vi "Do.vi"(8 "error in":errorcluster, 10 "Actor in":refnum<class "Actor.lvclass">, 11 "DS Reply Msg in":refnum<class "Reply Msg DataSocket Simple.lvclass">) -> (0 "error out":errorcluster, 2 "Actor out":refnum<class "Actor.lvclass">)   [LabVIEW 2023, in "Reply Msg DataSocket Simple.lvclass"]
uses:
  Reply Msg DataSocket Simple.lvclass
  <vilib>/ActorFramework/Actor/Actor.lvclass
  Reply Msg DataSocket Simple.lvclass/Reply Msg DataSocket Simple.ctl
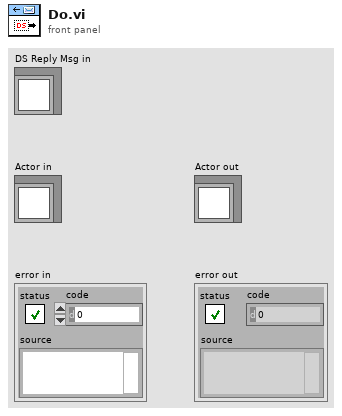
[diagram p1: front panel]
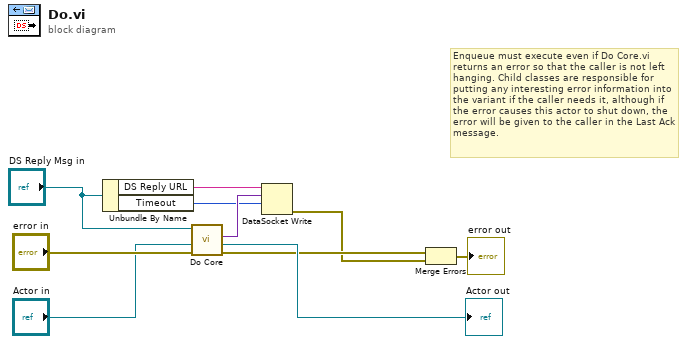
[diagram p0: block diagram]
diagram:
  # "Enqueue must execute even if Do Core.vi returns an error so that the caller is not left hanging. Child classes are responsible for putting any interesting error information into the variant if the caller needs it, although if the error causes this actor to shut down, the error will be given to the caller in the Last Ack message."
  n1 = Unbundle By Name("DS Reply Msg in") -> ("DS Reply URL"=w4:string, "Timeout"=w1:i32)
  n2 = call-dynamic "Do Core.vi"("error in"="error in", "Actor in"="Actor in", "DS Reply Msg in"="DS Reply Msg in") -> ("error out"=w6:errorcluster, "Actor out"=→"Actor out":refnum<class "Actor.lvclass">, "Reply"=w2:variant)  [unwired: 6 in]
  n3 = DataSocket Write(9:w1, 10:w2, 11:w4) -> (0:w3:errorcluster)  [unwired: 1 in, 2 out]
  n4 = Merge Errors(w6, w3) -> (→"error out":errorcluster)
